vi "Configure Prune All.vi"(8 "Error In":errorcluster, 11 "Prune All":bool) -> (0 "Error Out":errorcluster)   [LabVIEW 2018, in "Toolkit.lvlib"]
doc: "Sets the flag to prune, i.e. delete, all files greater than the maximum file count. For example, if there are ten (10) files on disk, and the maximum file count is set to two (2) and this is <B>true</B>, then the eight (8) oldest log files will be deleted. If this <B>false</B>, then the eight (8) oldest log files will remain on disk, but rollover of two files will continue. The default is <B>false</B> because this was the default behavior before the addition of this feature."
uses:
  Toolkit.lvlib
  Support/File/Action.ctl
  Support/File/File.lvlib
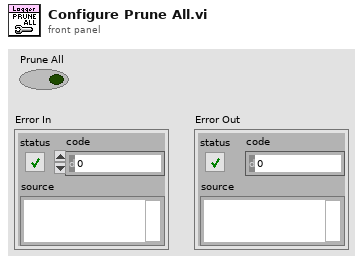
[diagram p1: front panel]
types:
  T1 = typedef "Toolkit.lvlib/File.lvlib/Action.ctl" = enum16{"Initialize", "Set Maximum File Size", "Set Maximum File Count", "Set Root Folder", "Set Enable Calendar Folder Tree", "Set File Extension", "Set Prune All", "Start", "Write", "Stop", "Shutdown"}
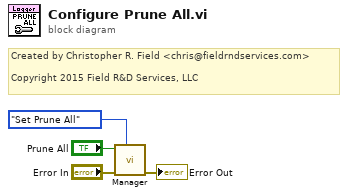
[diagram p0: block diagram]
diagram:
  # "Created by Christopher R. Field <chris@fieldrndservices.com>\n\nCopyright 2015 Field R&D Services, LLC"
  n1 = call "Manager.vi"("Action"=Action."Set Prune All", "Error In"="Error In", "Set Value"="Prune All") -> ("Error Out"=→"Error Out":errorcluster)  [unwired: 8 in]
